vi "整合-测量信息至列表框-网络版.vi"(9 "MCListbox引用句柄":refnum<vi>, 11 "探头属性数组":T2[](array[typedef])) -> (0 "测量状态":T1)   [LabVIEW 2017]
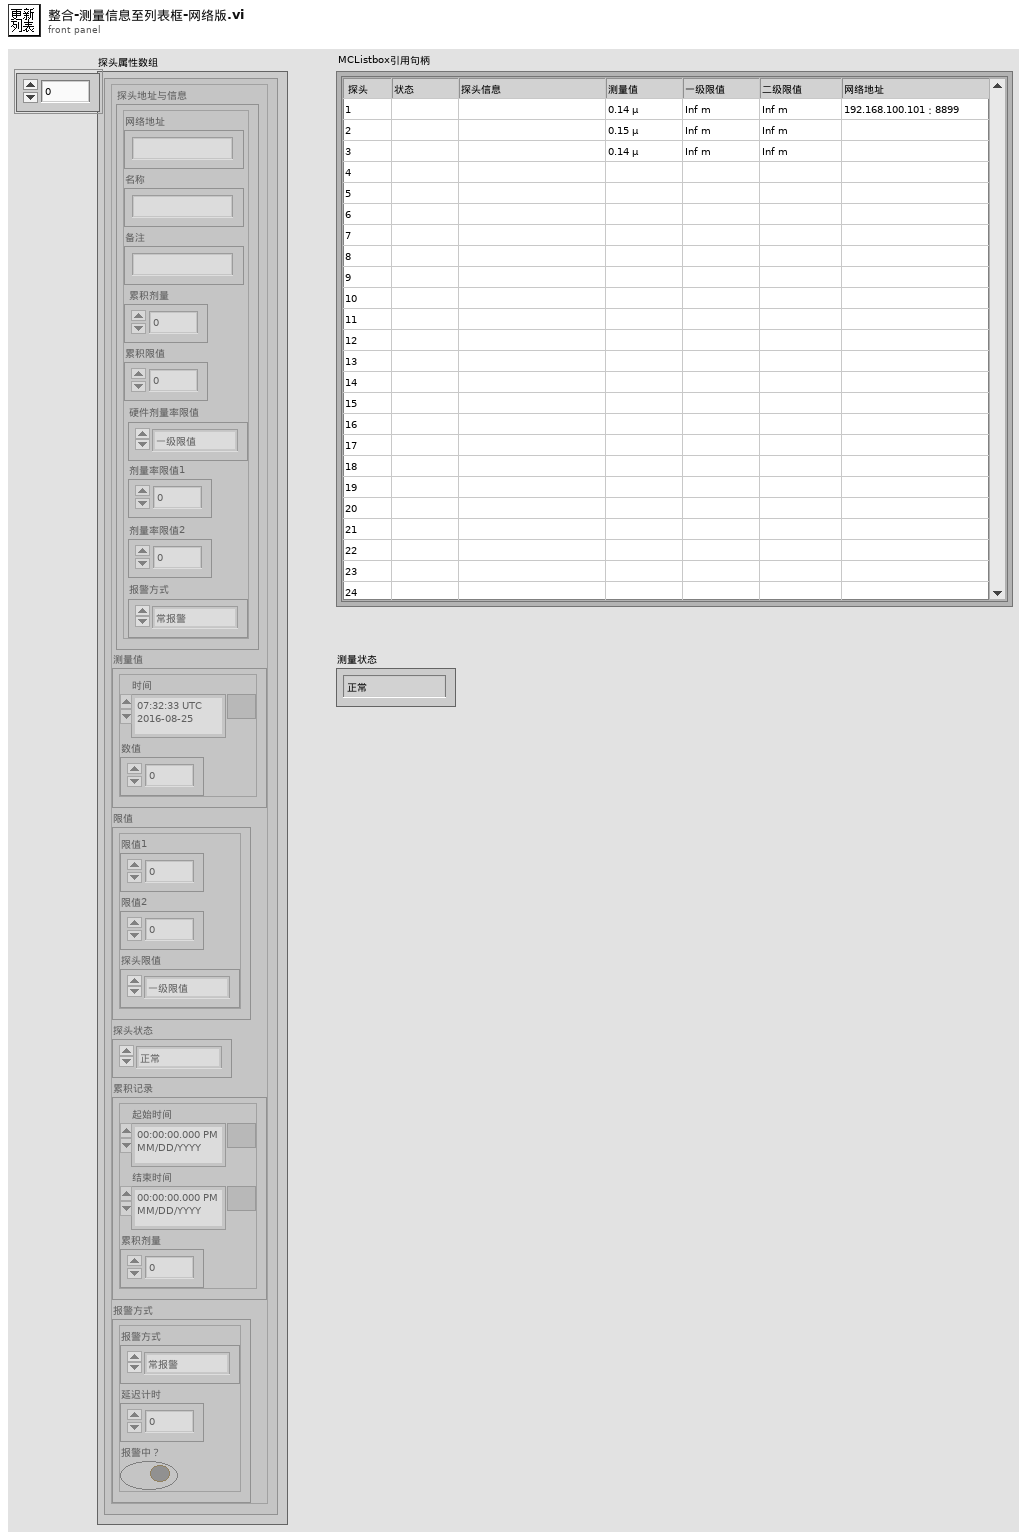
[diagram p1: front panel]
types:
  T1 = typedef "测量状态.ctl" = enum16{"正常", "一级报警", "二级报警", "累积报警", "有掉线"}
  T2 = typedef "探头属性.ctl" = cluster{"探头地址与信息":T3, "测量值":T6, "限值":T7, "探头状态":T8, "累积记录":T9, "报警方式":T10}
  T3 = typedef "探测器信息.ctl" = cluster{"网络地址":string, "名称":string, "备注":string, "累积剂量":dbl, "累积限值":dbl, "硬件剂量率限值":T4, "剂量率限值1":dbl, "剂量率限值2":dbl, "报警方式":T5}
  T4 = typedef "探头剂量率限值选择.ctl" = enum16{"一级限值", "二级限值"}
  T5 = typedef "报警方式选择.ctl" = enum16{"常报警", "自动静音", "手动静音"}
  T6 = typedef "测量值.ctl" = cluster{"时间":timestamp, "数值":dbl}
  T7 = typedef "剂量率限值.ctl" = cluster{"限值1":dbl, "限值2":dbl, "探头限值":T4}
  T8 = typedef "探头状态.ctl" = enum16{"正常", "离线", "禁用", "一级报警", "二级报警", "累积报警"}
  T9 = typedef "单条累积记录.ctl" = cluster{"起始时间":timestamp, "结束时间":timestamp, "累积剂量":dbl}
  T10 = typedef "报警方式.ctl" = cluster{"报警方式":T5, "延迟计时":u16, "报警中？":bool}
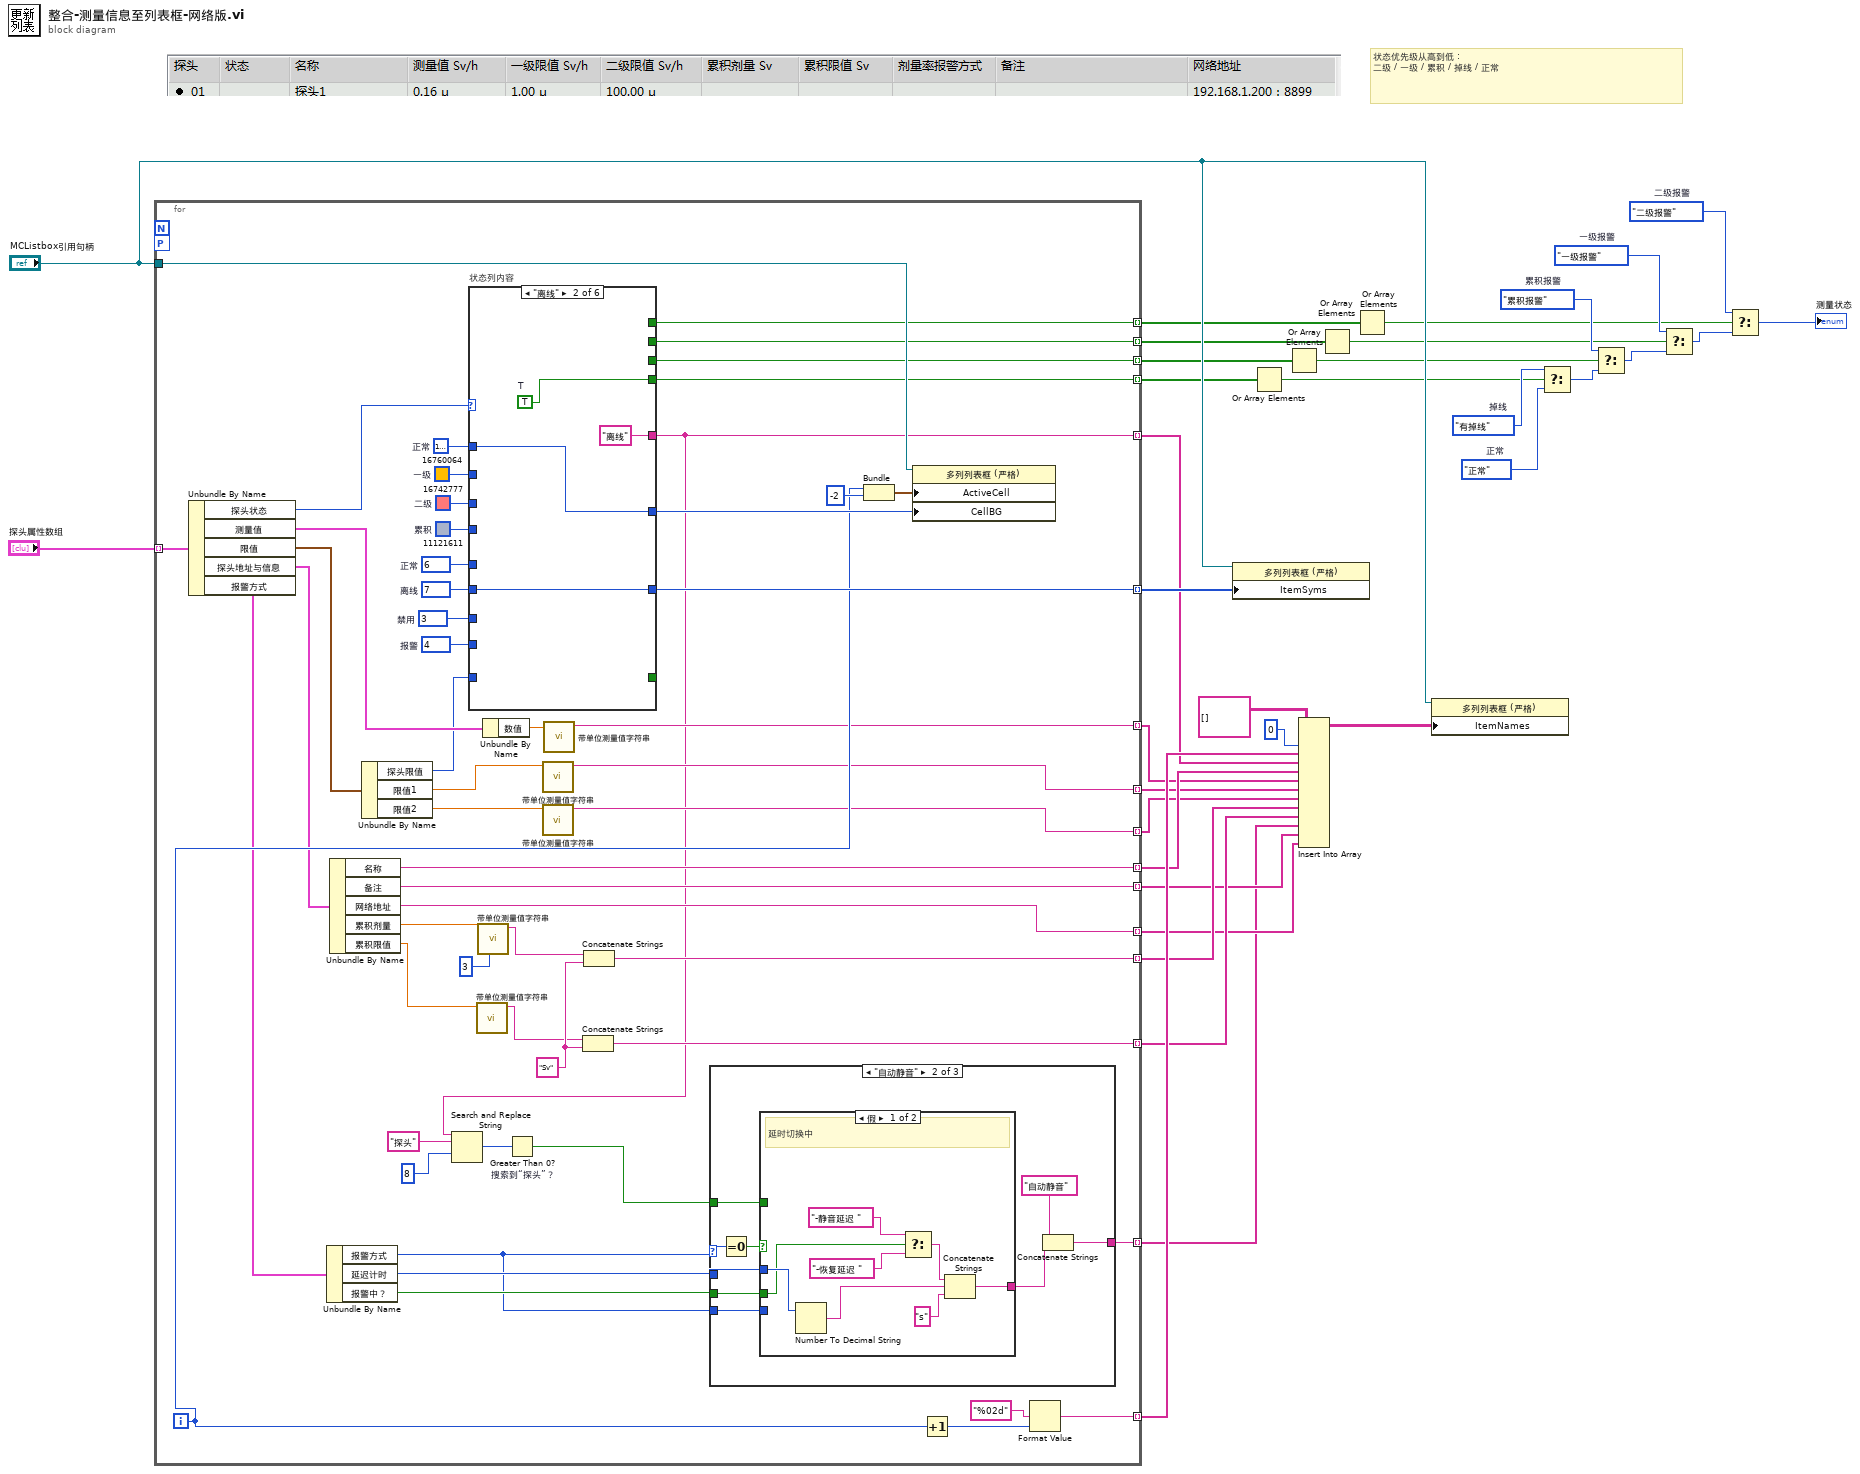
[diagram p0: block diagram]
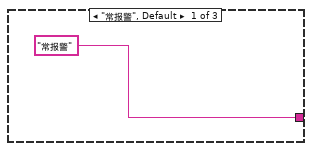
[diagram p2: hidden frame]
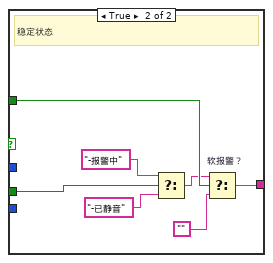
[diagram p3: hidden frame]
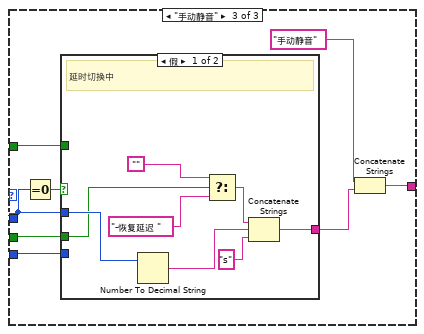
[diagram p4: hidden frame]
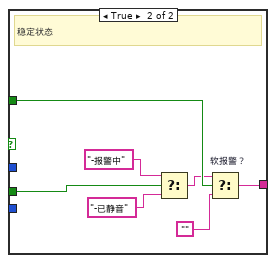
[diagram p5: hidden frame]
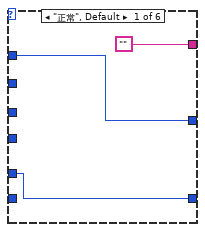
[diagram p6: hidden frame]
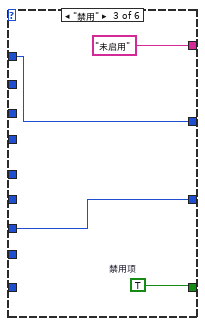
[diagram p7: hidden frame]
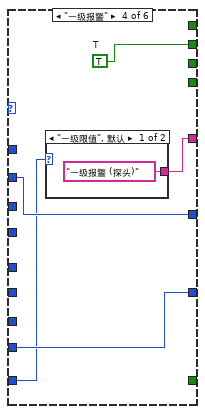
[diagram p8: hidden frame]
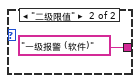
[diagram p9: hidden frame]
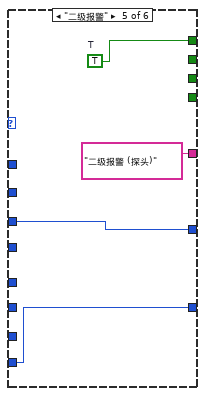
[diagram p10: hidden frame]
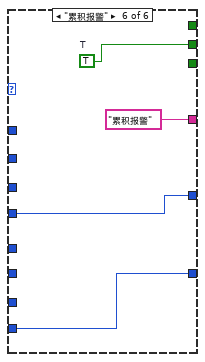
[diagram p11: hidden frame]
diagram:
  w12 = 测量状态."累积报警"  # 累积报警
  w14 = 测量状态."二级报警"  # 二级报警
  w13 = 测量状态."一级报警"  # 一级报警
  w16 = 测量状态."有掉线"  # 掉线
  w15 = 测量状态."正常"  # 正常
  # "状态优先级从高到低 :\n二级 / 一级 / 累积 / 掉线 / 正常"
  n1 = for {
    workers-P: _ -> [_]
    tunnel: "探头属性数组" -> [w88] mode=indexing
    tunnel: [w79] -> w33 mode=indexing
    tunnel: "MCListbox引用句柄" -> [w75]
    tunnel: [w73] -> w30 mode=indexing
    tunnel: [w50] -> w29 mode=indexing
    tunnel: [w60] -> w20 mode=indexing
    tunnel: [w57] -> w28 mode=indexing
    tunnel: [w69] -> w27 mode=indexing
    tunnel: [w65] -> w26 mode=indexing
    tunnel: [w64] -> w25 mode=indexing
    tunnel: [w59] -> w22 mode=indexing
    tunnel: [w58] -> w21 mode=indexing
    tunnel: [w56] -> w19 mode=indexing
    tunnel: [w45] -> w18 mode=indexing
    tunnel: [w43] -> w17 mode=indexing
    tunnel: [w42] -> w9 mode=indexing
    tunnel: [w41] -> w10 mode=indexing
    tunnel: [w40] -> w11 mode=indexing
    i -> [w74]
    w44 = "Sv" ("字符串")
    w61 = u32 11121611  # 累积
    w81 = 4  # 报警
    w82 = 3  # 禁用
    w83 = 7  # 离线
    w84 = 6  # 正常
    w85 = u32 16742777  # 二级
    w86 = u32 16760064  # 一级
    w87 = u32 16777226  # 正常
    n2 = Unbundle By Name(w88) -> ("探头状态"=w63:T8, "测量值"=w71:T6, "限值"=w66:T7, "探头地址与信息"=w72:T3, "报警方式"=w55:T10)
    n3 = Unbundle By Name(w55) -> ("报警方式"=w47:T5, "延迟计时"=w49:u16, "报警中？"=w48:bool)
    n4 = Unbundle By Name(w72) -> ("名称"=w57:string, "备注"=w56:string, "网络地址"=w60:string, "累积剂量"=w39:dbl, "累积限值"=w36:dbl)
    n5 = Unbundle By Name(w66) -> ("探头限值"=w54:T4, "限值1"=w67:dbl, "限值2"=w68:dbl)
    n6 = case "状态列内容" shown="\"离线\"" w63 {
      tunnel: ["" "离线" "未启用" w148 "二级报警 (探头)" "累积报警"] -> w50
      tunnel: w87 -> [w137 w141 w145 _ _ _]
      tunnel: w86 -> [_ _ _ w151 _ _]
      tunnel: w85 -> [_ _ _ _ w156 _]
      tunnel: [w137 w141 w145 w151 w156 w160] -> w76
      tunnel: w84 -> [w136 _ _ _ _ _]
      tunnel: w83 -> [_ w140 _ _ _ _]
      tunnel: w82 -> [_ _ w144 _ _ _]
      tunnel: [w136 w140 w144 w150 w155 w159] -> w79
      tunnel: w81 -> [_ _ _ w150 w155 w159]
      tunnel: [_ _ w143 _ _ _] -> _
      tunnel: w61 -> [_ _ _ _ _ w160]
      tunnel: w54 -> [_ _ _ w149 _ _]
      tunnel: [_ _ _ _ w154 _] -> w43
      tunnel: [_ _ _ w147 _ _] -> w42
      tunnel: [_ _ _ _ _ w158] -> w41
      tunnel: [_ w139 _ _ _ _] -> w40
      frame "正常", Default {
      }
      frame "离线" {
        w139 = TRUE  # T
      }
      frame "禁用" {
        w143 = TRUE  # 禁用项
      }
      frame "一级报警" {
        w147 = TRUE  # T
        n7 = case shown="\"一级限值\", 默认" w149 {
          tunnel: ["一级报警 (探头)" "一级报警 (软件)"] -> w148
          frame "一级限值", Default {
          }
          frame "二级限值" {
          }
        }
      }
      frame "二级报警" {
        w154 = TRUE  # T
      }
      frame "累积报警" {
        w158 = TRUE  # T
      }
    }
    n8 = Search and Replace String(input string=w50, search string="探头" ("正则表达式"), offset=8 ("偏移量(0)")) -> (number of replacements=w53:i32)  [unwired: 5 in, 3 out]
    n9 = call "带单位测量值字符串.vi"("测量值"=w36) -> ("结果"=w35:string)  [unwired: 10 in]
    n10 = call "带单位测量值字符串.vi"("精度(2)"=i16 3 ("精度(6)"), "测量值"=w39) -> ("结果"=w38:string)  [unwired: 9 in]
    n11 = Unbundle By Name(w71) -> ("数值"=w70:dbl)
    n12 = Greater Than 0? "搜索到“探头”？"(x=w53) -> (x > 0?=w46:bool)
    n13 = call "带单位测量值字符串.vi"("测量值"=w67) -> ("结果"=w65:string)  [unwired: 10 in]
    n14 = call "带单位测量值字符串.vi"("测量值"=w68) -> ("结果"=w64:string)  [unwired: 10 in]
    n15 = call "带单位测量值字符串.vi"("测量值"=w70) -> ("结果"=w69:string)  [unwired: 10 in]
    n16 = Concatenate Strings(w35, w44) -> (w58:string)
    n17 = Concatenate Strings(w38, w44) -> (w59:string)
    n18 = case shown="\"自动静音\"" w47 {
      tunnel: w48 -> [_ w96 w115]
      tunnel: w49 -> [_ w95 w116]
      tunnel: w47 -> [_ w93 w114]
      tunnel: ["常报警" w92 w113] -> w45
      tunnel: w46 -> [_ w90 w117]
      frame "常报警", Default {
      }
      frame "自动静音" {
        n19 = Equal To 0?(x=w95) -> (x = 0?=w97:bool)
        n20 = case shown="假" w97 {
          tunnel: w96 -> [w98 w112]
          tunnel: w95 -> [w103 _]
          tunnel: [w99 w106] -> w94
          tunnel: w93 -> [_ _]
          tunnel: w90 -> [_ w109]
          frame False {
            # "延时切换中"
            n21 = Number To Decimal String(number=w103) -> (decimal integer string=w101:string)  [unwired: 1 in]
            n22 = Select(t="-静音延迟 ", s=w98, f="-恢复延迟 ") -> (s? t:f=w102:string)
            n23 = Concatenate Strings(w102, w101, "s") -> (w99:string)
          }
          frame True {
            # "稳定状态"
            n24 = Select(t="-报警中", s=w112, f="-已静音") -> (s? t:f=w108:string)
            n25 = Select "软报警？"(t=w108, s=w109, f="") -> (s? t:f=w106:string)
          }
        }
        n26 = Concatenate Strings("自动静音", w94) -> (w92:string)
      }
      frame "手动静音" {
        n27 = Equal To 0?(x=w116) -> (x = 0?=w120:bool)
        n28 = case shown="假" w120 {
          tunnel: w115 -> [w121 w135]
          tunnel: w116 -> [w126 _]
          tunnel: [w122 w129] -> w119
          tunnel: w114 -> [_ _]
          tunnel: w117 -> [_ w132]
          frame False {
            # "延时切换中"
            n29 = Number To Decimal String(number=w126) -> (decimal integer string=w124:string)  [unwired: 1 in]
            n30 = Select(t="", s=w121, f="-恢复延迟 ") -> (s? t:f=w125:string)
            n31 = Concatenate Strings(w125, w124, "s") -> (w122:string)
          }
          frame True {
            # "稳定状态"
            n32 = Select(t="-报警中", s=w135, f="-已静音") -> (s? t:f=w131:string)
            n33 = Select "软报警？"(t=w131, s=w132, f="") -> (s? t:f=w129:string)
          }
        }
        n34 = Concatenate Strings("手动静音", w119) -> (w113:string)
      }
    }
    n35 = Bundle(w74, -2) -> (w77:cluster{i32, i32})  [unwired: 1 in]
    n36 = property class="多列列表框 (严格)"(reference=w75, "ActiveCell"=w77, "CellBG"=w76) -> ()  [unwired: 1 in, 2 out]
    n37 = Increment(x=w74) -> (x+1=w62:i32)
    n38 = Format Value(format string="%02d" ("格式字符串"), value (0)=w62) -> (output string=w73:string)  [unwired: 1 in]
  }
  n39 = property class="多列列表框 (严格)"(reference="MCListbox引用句柄", "ItemSyms"=w33) -> ()  [unwired: 1 in, 2 out]
  n40 = Or Array Elements(Boolean array=w11) -> (logical OR=w1:bool)
  n41 = Or Array Elements(Boolean array=w10) -> (logical OR=w2:bool)
  n42 = Insert Into Array(array=string[][] [] ("十进制整型字符串"), index (col)=0 ("禁用的索引 (列)"), new element #1=w30, new element #2=w29, new element #3=w28, new element #4=w27, new element #5=w26, new element #6=w25, new element #7=w22, new element #8=w21, new element #9=w18, new element #10=w19, new element #11=w20) -> (w24:string[][])  [unwired: 1 in]
  n43 = Or Array Elements(Boolean array=w9) -> (logical OR=w3:bool)
  n44 = Or Array Elements(Boolean array=w17) -> (logical OR=w4:bool)
  n45 = property class="多列列表框 (严格)"(reference="MCListbox引用句柄", "ItemNames"=w24) -> ()  [unwired: 1 in, 2 out]
  n46 = Select(t=w16, s=w1, f=w15) -> (s? t:f=w8:T1)
  n47 = Select(t=w12, s=w2, f=w8) -> (s? t:f=w7:T1)
  n48 = Select(t=w13, s=w3, f=w7) -> (s? t:f=w6:T1)
  n49 = Select(t=w14, s=w4, f=w6) -> (s? t:f=→"测量状态":T1)
